vi "Main.vi"() -> ()   [LabVIEW 2021, in "Game of Life.lvlib"]
doc: "This template is for the Queued Message Handler design pattern.\n\nThe Event Handling Loop generates messages based on user interface actions.\n\nThe Message Handling Loop processes messages generated by the Event Handling Loop, or by other messages. The messages are string values, so new messages can be added easily to the Message Cases case structure in the Message Handling Loop. Each message cluster can also provide an optional value for Message Data, which is a variant that can be converted to whatever message-specific data is required."
uses:
  Game of Life.lvlib
  <vilib>/Plug-In SDKs/InstrumentStudio SDK/InstrumentStudioPluginSDK.lvlibp/Plugin Events Enum.ctl
  controls/Data.ctl
  controls/Configuration.ctl
  controls/Game of Life.ctl
  a2cd5499-92a9-455c-b0f9-1db12e3f6067.vi
  aef85ed4-6d5b-4a62-8cd4-232f16e6ae51.vi
  a2cd5499-92a9-455c-b0f9-1db12e3f6067.vi/6651a77e-856e-4bcd-af5a-c0c13b264cc1.vi
  aef85ed4-6d5b-4a62-8cd4-232f16e6ae51.vi/331b549c-fcf8-43d9-8a1e-5b3c0091a99c.vi
  <vilib>/JDP Science/JSONtext/JSON text to Variant.vi
  <vilib>/Utility/error.llb/Error Cluster From Error Code.vi
  <vilib>/JDP Science/JSONtext/Variant to JSON Text.vi
  <vilib>/JDP Science/JSONtext/LVClass Serializer/JSONtext LVClass Serializer.lvclass
  <vilib>/ErrorRing/Error Ring.xnode
  <vilib>/Plug-In SDKs/InstrumentStudio SDK/InstrumentStudioPluginSDK.lvlibp/Plugin Session.lvclass
  <vilib>/Plug-In SDKs/InstrumentStudio SDK/InstrumentStudioPluginSDK.lvlibp
panel:
  in  "Tab Control":enum32{"Game Panel", "Events"}(tab)
  in  "Start":bool
  out "game of life":T1(graph)
  out "generation":u32 caption="Generation"
  in  "update interval":u32=250 caption="Update interval (msec)" min=50
  in  "height":u32=100 caption="Board height" min=10
  in  "width":u32=100 caption="Board width" min=10
  in  "Log Events?":bool
  out "Event Record":i32(listbox)
  in  "Session Id":u64
  # "Enable Logging: Check this box to generate a log file and save the event record."
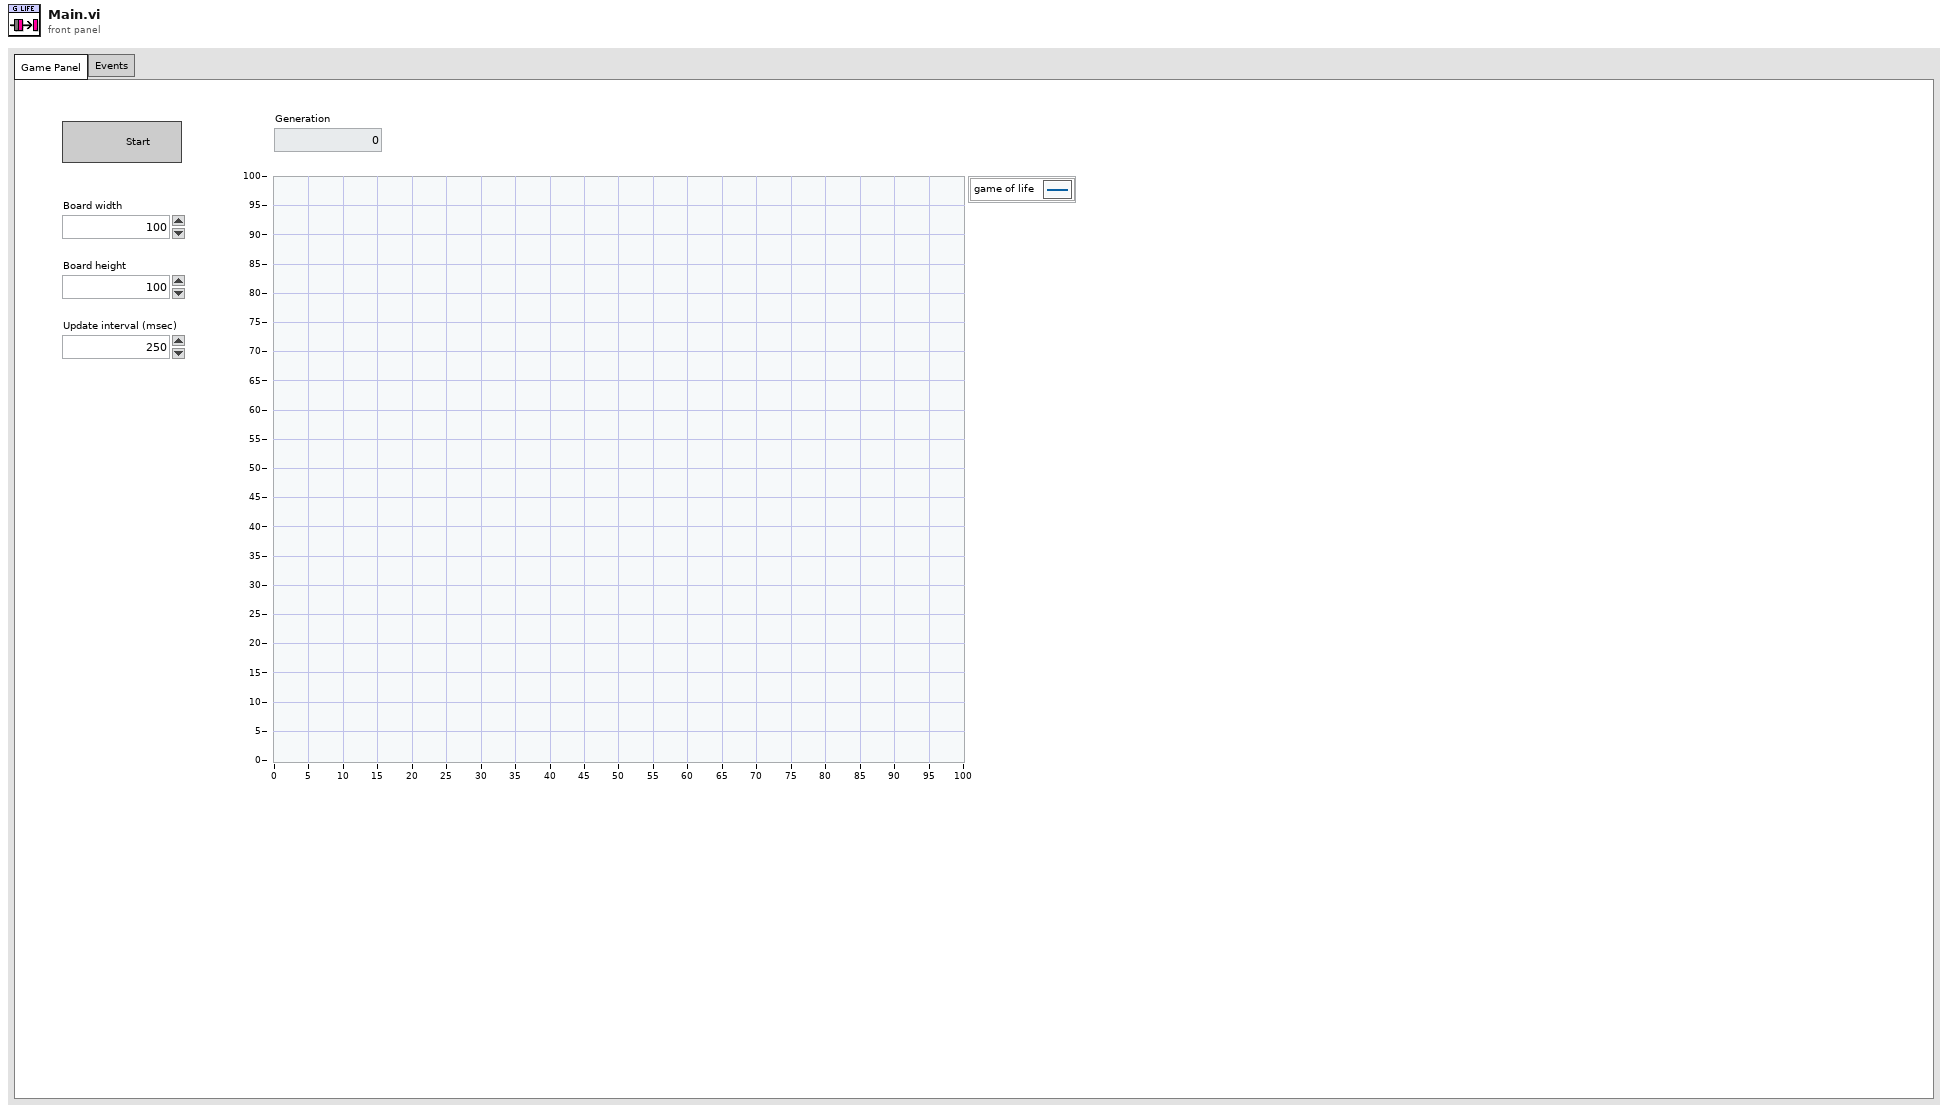
[diagram p1: front panel]
types:
  T1 = typedef "Game of Life.lvlib/Game of Life.ctl" = cluster{"x_data":dbl[], "y_data":dbl[]}
  T2 = typedef "Game of Life.lvlib/Data.ctl" = cluster{"Configuration":T3, "Generation":u32, "Run?":bool, "Cells":bool[][], "Log Events?":bool}
  T3 = typedef "Game of Life.lvlib/Configuration.ctl" = cluster{"Height":u32, "Width":u32, "Update Interval":u32}
  T4 = typedef "InstrumentStudioPluginSDK.lvlibp/Plugin Events Enum.ctl" = enum16{"Shutdown", "Project Saved", "Stop All Outputs"}
  T5 = typedef "InstrumentStudioPluginSDK.lvlibp/Event Registration Refnum.ctl" = refnum<event-registration>
  T6 = typedef "Game of Life.lvlib/All Message Queues.ctl" = cluster{"UI":refnum<queue>}
  T7 = cluster{"Event Refnum":T5, "Event Registration Refnum":refnum<event-registration>}
  T8 = enum8{"Enabled", "Disabled", "Disabled and Grayed Out"}
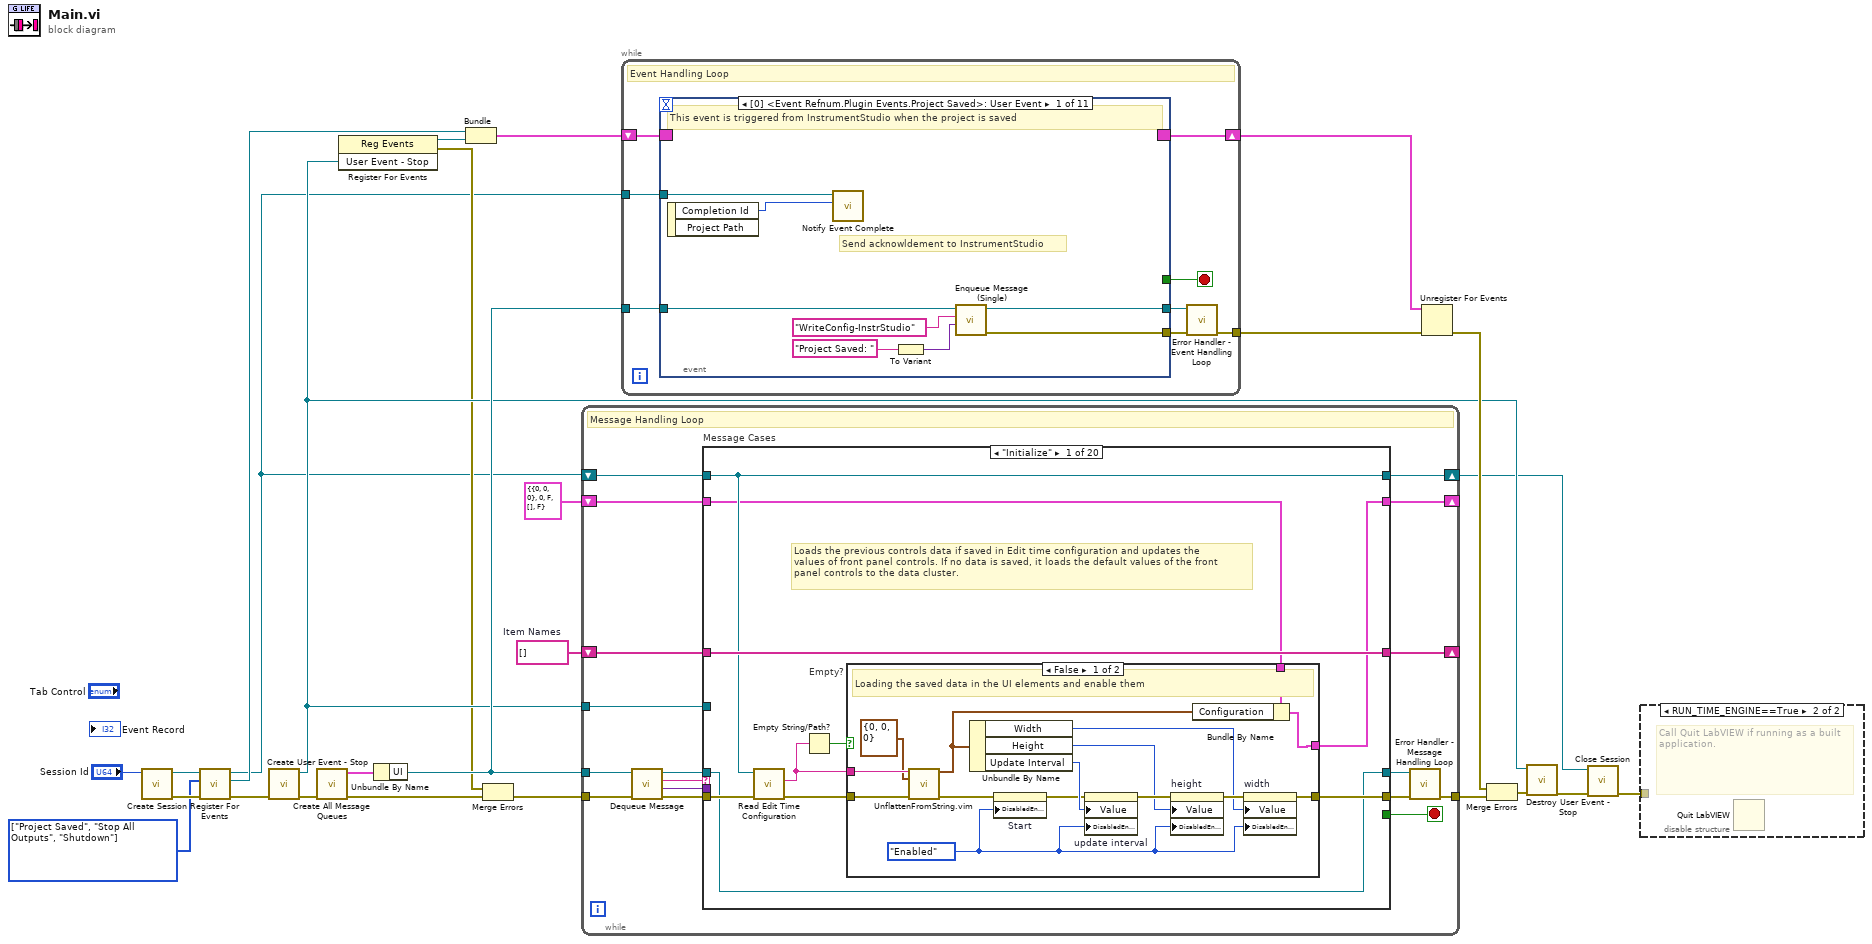
[diagram p0: block diagram]
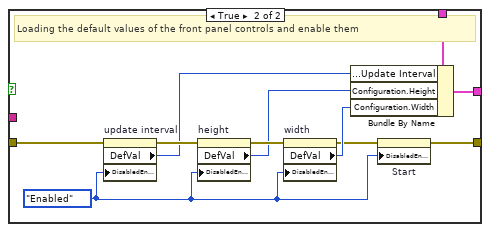
[diagram p3: hidden frame]
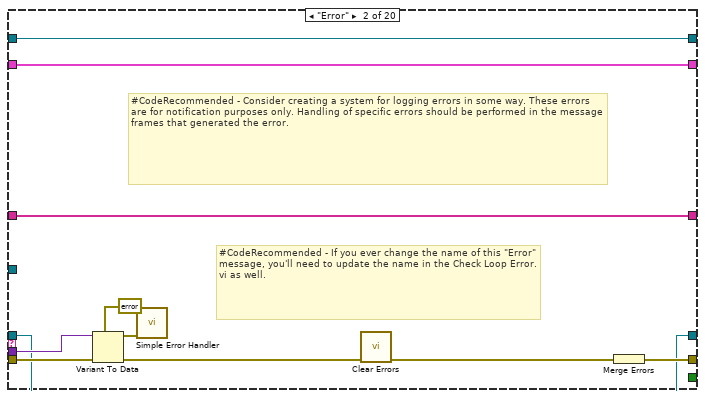
[diagram p4: hidden frame]
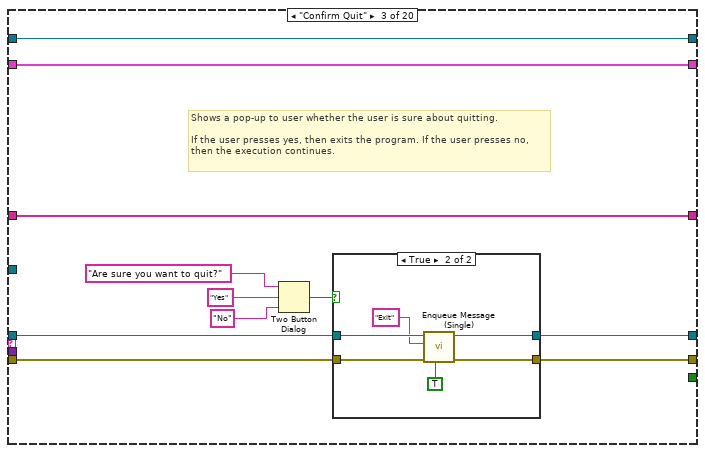
[diagram p5: hidden frame]
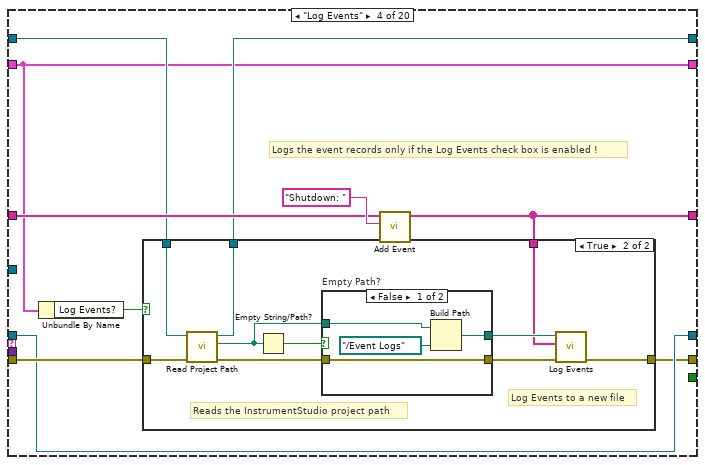
[diagram p7: hidden frame]
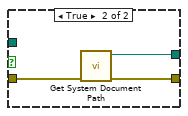
[diagram p9: hidden frame]
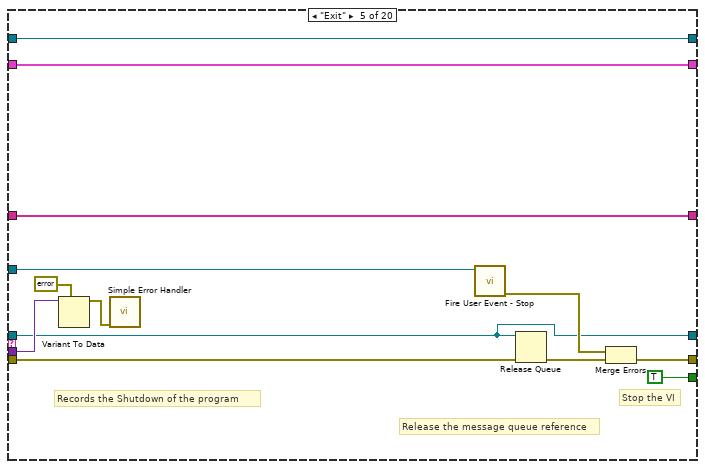
[diagram p10: hidden frame]
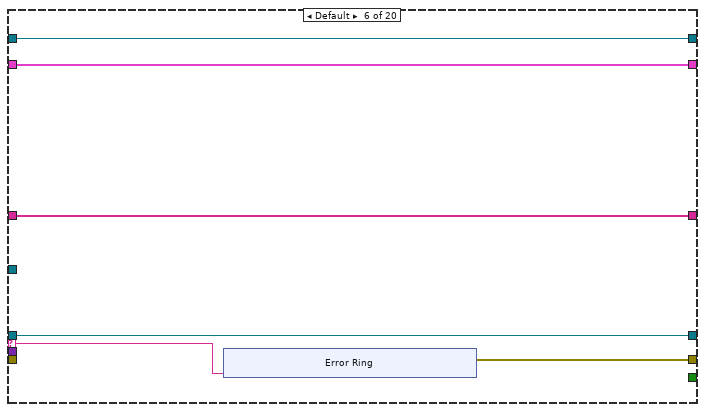
[diagram p11: hidden frame]
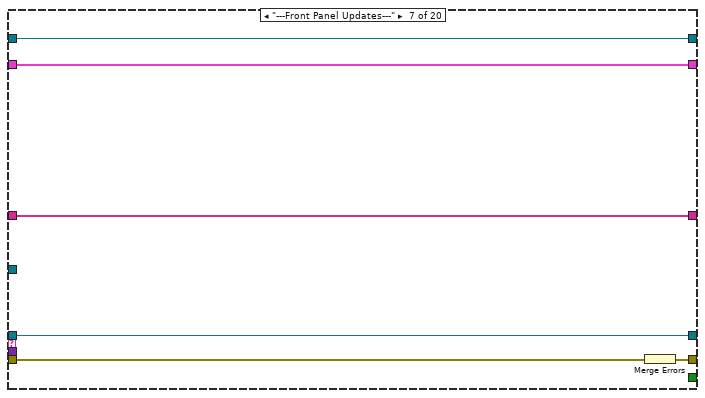
[diagram p12: hidden frame]
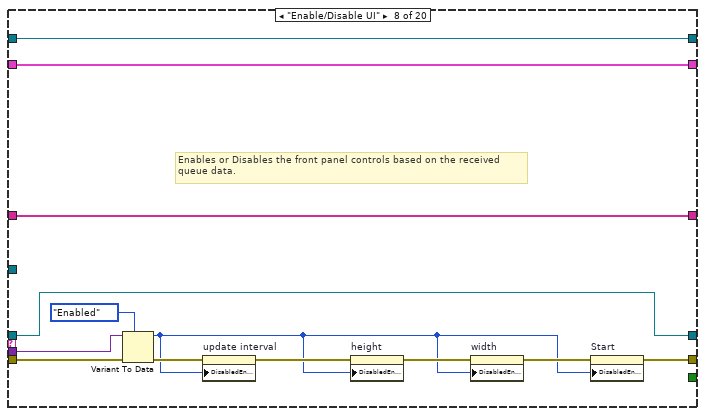
[diagram p13: hidden frame]
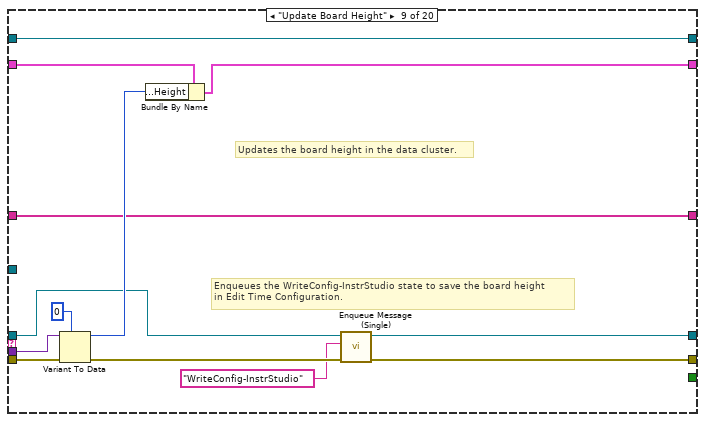
[diagram p14: hidden frame]
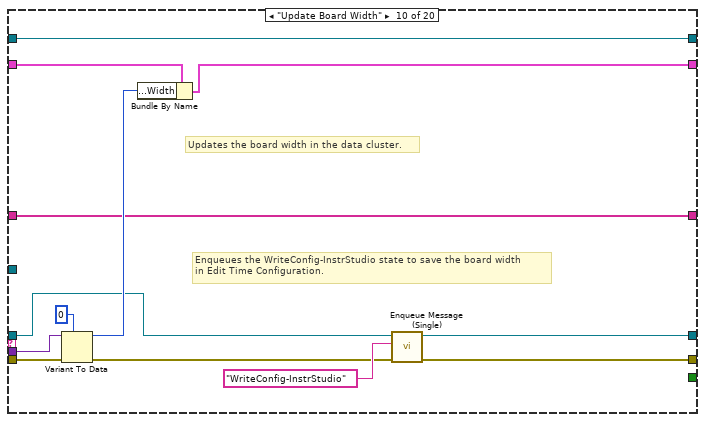
[diagram p15: hidden frame]
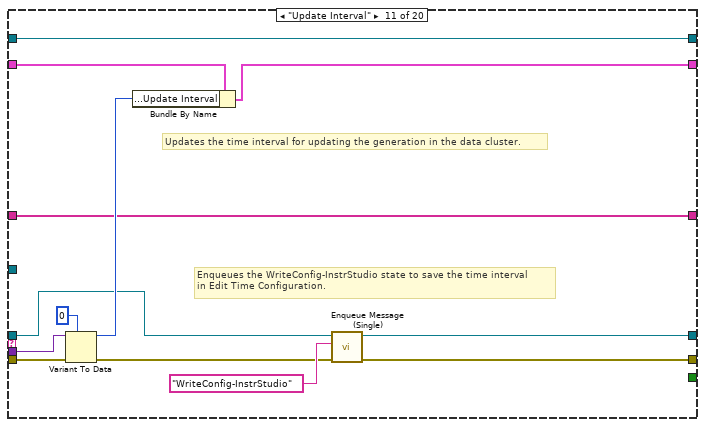
[diagram p16: hidden frame]
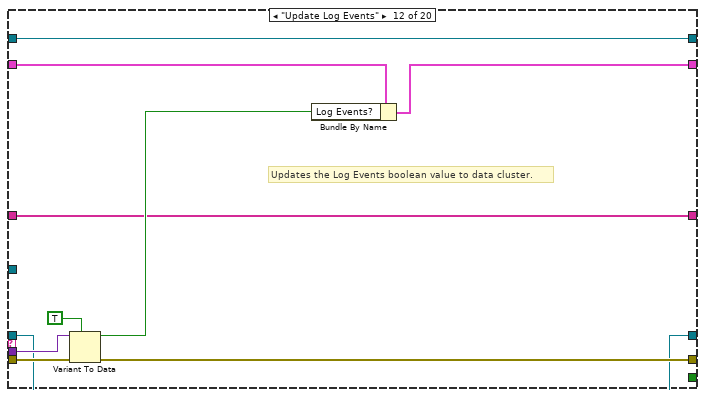
[diagram p17: hidden frame]
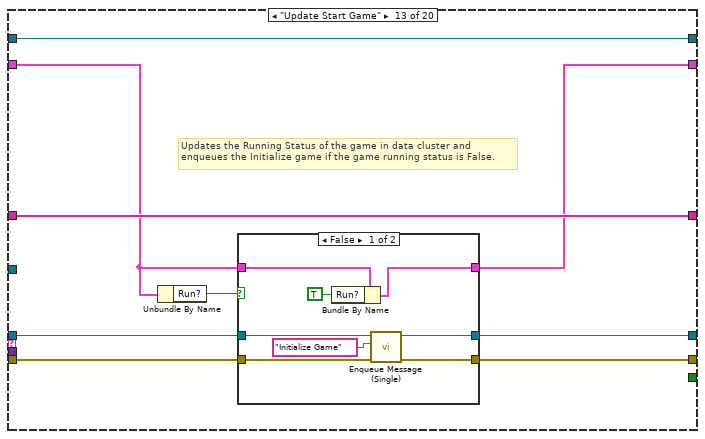
[diagram p18: hidden frame]
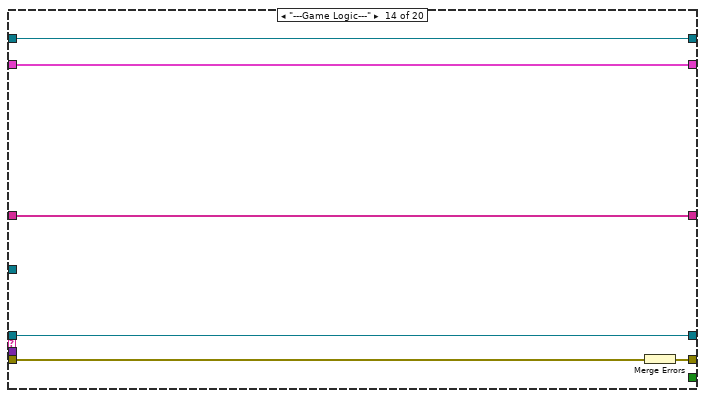
[diagram p20: hidden frame]
diagram:
  w1 = string[] []  # Item Names
  w10 = T4[] [enum."Project Saved", enum."Stop All Outputs", enum."Shutdown"] items=["Shutdown", "Project Saved", "Stop All Outputs"] ("Events To Register")
  n1 = call <vilib>:"Create Session.vi"("Session Id"="Session Id") -> ("error out"=w13:errorcluster, "Session out"=w11:refnum<class "Plugin Session.lvclass">)  [unwired: 6 in, 3 out]
  n2 = call <vilib>:"Register For Events.vi"("error in (no error)"=w13, "Events To Register"=w10, "Session in"=w11) -> ("error out"=w12:errorcluster, "Event Refnum"=w7:T5, "Session out"=w3:refnum<class "Plugin Session.lvclass">)  [unwired: 6 in]
  n3 = call "Create User Event - Stop.vi"("error in (no error)"=w12) -> ("error out"=w22:errorcluster, "User Event - Stop"=w17:refnum<user-event>)  [unwired: 9 in]
  n4 = call "Create All Message Queues.vi"("error in (no error)"=w22) -> ("error out"=w26:errorcluster, "Message Queues out"=w25:T6)  [unwired: 9 in]
  n5 = register-events(w17) -> (reference out=w9:refnum<event-registration>, error out=w15:errorcluster)  [unwired: 2 in]
  n6 = Unbundle By Name(w25) -> ("UI"=w23:refnum<queue>)
  n7 = Bundle("Event Refnum"=w7, "Event Registration Refnum"=w9) -> (w8:T7)  [unwired: 1 in]
  n8 = Merge Errors(w15, w26) -> (w16:errorcluster)
  n9 = while {
    tunnel: w23 -> [w37]
    tunnel: w17 -> [w42]
    tunnel: w16 -> [w41]
    tunnel: [w35] -> w24
    shift-right: [w32] -> w6
    shift-left: w3 -> [w33]
    shift-right: [w31] -> _
    shift-left: T2 {"Configuration"={"Height"=0, "Width"=0, "Update Interval"=0}, "Generation"=0, "Run?"=FALSE, "Cells"=[], "Log Events?"=FALSE} ("Configuration") -> [w30]
    shift-right: [w28] -> _
    shift-left: w1 -> [w29]
    stop <- w43 stop-if-true
    # "Message Handling Loop"
    n10 = call "Dequeue Message.vi"("error in (no error)"=w41, "Message Queue"=w37) -> ("error out"=w40:errorcluster, "Message Data"=w38:variant, "Message"=w39:string, "dup Message Queue"=w36:refnum<queue>)  [unwired: 6 in]
    n11 = case "Message Cases" shown="\"Initialize\"" w39 {
      selector: w39 -> [_ _ _ _ _ w155 _ _ _ _ _ _ _ _ _ _ _ _ _ _]
      tunnel: w36 -> [w46 w80 w99 w114 w140 w151 w164 w171 w184 w197 w209 w226 w233 w252 w271 w284 w318 w334 w343 w355]
      tunnel: w40 -> [w49 w90 w101 w117 w139 _ w169 w175 w194 w207 w220 w229 w239 w257 w269 w289 w323 w336 w345 w354]
      tunnel: [w53 w85 w100 w113 w148 w156 w168 w177 w186 w196 w211 w230 w234 w256 w272 w285 w322 w332 w346 w361] -> w34
      tunnel: [_ _ _ _ TRUE _ _ _ _ _ _ _ _ _ _ _ _ _ _ _] -> w43
      tunnel: w38 -> [_ w89 _ _ w143 _ _ w174 w193 w206 w219 w228 _ _ _ _ _ _ _ w352]
      tunnel: w42 -> [_ _ _ _ w147 _ _ _ _ _ _ _ _ _ _ _ _ _ _ _]
      tunnel: w33 -> [w47 w84 w98 w115 w142 w154 w167 w182 w195 w208 w221 w231 w240 w255 w277 w290 w321 w340 w348 w363]
      tunnel: [w47 w84 w98 w116 w142 w154 w167 w182 w195 w208 w221 w231 w240 w255 w277 w290 w321 w340 w347 w362] -> w32
      tunnel: [w45 w83 w97 w111 w141 w153 w166 w181 w190 w204 w217 w225 w235 w254 w276 w278 w320 w338 w342 w356] -> w31
      tunnel: w30 -> [w44 w83 w97 w111 w141 w153 w166 w181 w189 w203 w216 w224 w236 w254 w275 w282 w320 w337 w342 w356]
      tunnel: w29 -> [w48 w81 w96 w118 w138 w152 w165 w170 w188 w201 w214 w222 w238 w253 w274 w288 w319 w328 w344 w353]
      tunnel: [w48 w81 w96 w112 w138 w152 w165 w170 w188 w201 w214 w222 w238 w253 w274 w288 w319 w329 w344 w357] -> w28
      tunnel: [w46 w80 w95 w114 w140 w151 w164 w171 w185 w198 w210 w226 w232 w252 w270 w281 w318 w330 w343 w355] -> w27
      frame "Initialize" {
        # "Loads the previous controls data if saved in Edit time configuration and updates the\nvalues of front panel controls. If no data is saved, it loads the default values of the front\npanel controls to the data cluster."
        # "Initialize - All initialization work should take place in this message, since other loops can potentially enqueue messages that execute immediately after this one."
        n12 = call <vilib>:"Read Edit Time Configuration.vi"("error in (no error)"=w49, "Session in"=w47) -> ("error out"=w50:errorcluster, "Edit Time Configuration"=w51:string)  [unwired: 7 in, 1 out]
        n13 = Empty String/Path?(string/path=w51) -> (empty?=w52:bool)
        n14 = case "Empty?" shown="False" w52 {
          tunnel: [w62 w70] -> w53
          tunnel: w50 -> [w67 w76]
          tunnel: w51 -> [w68 _]
          tunnel: w44 -> [w59 w79]
          tunnel: [w58 w74] -> w45
          frame False {
            w54 = T8."Enabled" ("Disabled")
            # "Loading the saved data in the UI elements and enable them"
            n15 = call "UnflattenFromString.vim"("Flattened Data"=w68, "Data Type"=T3 {"Height"=0, "Width"=0, "Update Interval"=0} ("Configuration"), "error in"=w67) -> ("Data Out"=w57:T3, "error out"=w56:errorcluster)  [unwired: 11 in]
            n16 = Unbundle By Name(w57) -> ("Width"=w61:u32, "Height"=w64:u32, "Update Interval"=w66:u32)
            n17 = property on="Start" class="Bool"(error in=w56, "DisabledEnum"=w54) -> (error out=w55:errorcluster)  [unwired: 1 in, 1 out]
            n18 = property on="update interval" class="DigNum (strict)"(error in=w55, "Value"=w66, "DisabledEnum"=w54) -> (error out=w65:errorcluster)  [unwired: 1 in, 1 out]
            n19 = property on="height" class="DigNum (strict)"(error in=w65, "Value"=w64, "DisabledEnum"=w54) -> (error out=w63:errorcluster)  [unwired: 1 in, 1 out]
            n20 = Bundle By Name(cluster=w59, "Configuration"=w57) -> (w58:T2)
            n21 = property on="width" class="DigNum (strict)"(error in=w63, "Value"=w61, "DisabledEnum"=w54) -> (error out=w62:errorcluster)  [unwired: 1 in, 1 out]
          }
          frame True {
            w69 = T8."Enabled" ("Disabled")
            # "Loading the default values of the front panel controls and enable them"
            n22 = property on="update interval" class="DigNum (strict)"(error in=w76, "DisabledEnum"=w69) -> (error out=w78:errorcluster, "DefVal"=w75:u32)  [unwired: 1 in, 1 out]
            n23 = property on="height" class="DigNum (strict)"(error in=w78, "DisabledEnum"=w69) -> (error out=w77:errorcluster, "DefVal"=w73:u32)  [unwired: 1 in, 1 out]
            n24 = property on="width" class="DigNum (strict)"(error in=w77, "DisabledEnum"=w69) -> (error out=w71:errorcluster, "DefVal"=w72:u32)  [unwired: 1 in, 1 out]
            n25 = Bundle By Name(cluster=w79, "Configuration.Update Interval"=w75, "Configuration.Height"=w73, "Configuration.Width"=w72) -> (w74:T2)
            n26 = property on="Start" class="Bool"(error in=w71, "DisabledEnum"=w69) -> (error out=w70:errorcluster)  [unwired: 1 in, 1 out]
          }
        }
      }
      frame "Error" {
        # "#CodeRecommended - If you ever change the name of this \"Error\" message, you'll need to update the name in the Check Loop Error.vi as well."
        # "#CodeRecommended - Consider creating a system for logging errors in some way. These errors are for notification purposes only. Handling of specific errors should be performed in the message frames that generated the error."
        # "Error - Display an error dialog. This message is sent by the \"Error Handler\" VIs at the end of other loops in this application."
        n27 = Variant To Data(error in=w90, type=errorcluster {"status"=FALSE, "code"=0, "source"=""} ("error constant"), Variant=w89) -> (data=w87:errorcluster, error out=w86:errorcluster)
        n28 = call <vilib>:"Simple Error Handler.vi"("error in (no error)"=w87) -> ()  [unwired: 4 in, 5 out]
        n29 = call <vilib>:"Clear Errors.vi"("error in (no error)"=w86) -> ("error out"=w82:errorcluster)  [unwired: 5 in, 1 out]
        n30 = Merge Errors(w82) -> (w85:errorcluster)
      }
      frame "Confirm Quit" {
        # "Shows a pop-up to user whether the user is sure about quitting. \n\nIf the user presses yes, then exits the program. If the user presses no,\nthen the execution continues."
        # "Confirm Quit - Message that can confirm whether or not the user wants to exit the application."
        n31 = Two Button Dialog(message="Are sure you want to quit?", 1:"No" ("F button name (\"Cancel\")"), 2:"Yes" ("T button name (\"OK\")")) -> (T button?=w91:bool)
        n32 = case shown="True" w91 {
          tunnel: w101 -> [w102 w109]
          tunnel: [w102 w108] -> w100
          tunnel: w99 -> [w103 w107]
          tunnel: [w103 w104] -> w95
          frame False {
          }
          frame True {
            n33 = call "Enqueue Message (Single).vi"("Priority Message? (F)"=TRUE, "error in (no error)"=w109, "Message"="Exit", "Message Queue"=w107) -> ("error out"=w108:errorcluster, "dup Message Queue"=w104:refnum<queue>)  [unwired: 6 in]
          }
        }
      }
      frame "Log Events" {
        # "Logs the event records only if the Log Events check box is enabled !"
        n34 = Unbundle By Name(w111) -> ("Log Events?"=w110:bool)
        n35 = call "Add Event.vi"("Event Tag"="Shutdown: ", "Item Names in"=w118) -> ("Item Names out"=w112:string[])  [unwired: 9 in]
        n36 = case shown="True" w110 {
          tunnel: w117 -> [w121 w131]
          tunnel: [w120 w130] -> w116
          tunnel: w115 -> [w120 w129]
          tunnel: [w121 w124] -> w113
          tunnel: w112 -> [_ w122]
          frame False {
          }
          frame True {
            # "Log Events to a new file"
            # "Reads the InstrumentStudio project path"
            n37 = call <vilib>:"Read Project Path.vi"("error in (no error)"=w131, "Session in"=w129) -> ("error out"=w127:errorcluster, "Project Path"=w126:path, "Session out"=w130:refnum<class "Plugin Session.lvclass">)  [unwired: 7 in]
            n38 = Empty String/Path?(string/path=w126) -> (empty?=w128:bool)
            n39 = case "Empty Path?" shown="False" w128 {
              tunnel: w127 -> [w135 w136]
              tunnel: w126 -> [w134 _]
              tunnel: [w132 w137] -> w125
              tunnel: [w135 w136] -> w123
              frame False {
                n40 = Build Path(base path=w134, name or relative path=path "../Event Logs") -> (appended path=w132:path)
              }
              frame True {
                n41 = call "Get System Document Path.vi"() -> ("Public Path"=w137:path)  [unwired: 11 in]
              }
            }
            n42 = call "Log Events.vi"("error in"=w123, "Item Names"=w122, "Event Folder Path"=w125) -> ("error out"=w124:errorcluster)  [unwired: 8 in]
          }
        }
      }
      frame "Exit" {
        # "Records the Shutdown of the program"
        # "Stop the VI"
        # "Release the message queue reference"
        # "Exit - Exit the application."
        n43 = Variant To Data(type=errorcluster {"status"=FALSE, "code"=0, "source"=""} ("error constant"), Variant=w143) -> (data=w144:errorcluster)  [unwired: 1 in, 1 out]
        n44 = call <vilib>:"Simple Error Handler.vi"("error in (no error)"=w144) -> ()  [unwired: 4 in, 5 out]
        n45 = call "Fire User Event - Stop.vi"("User Event - Stop"=w147) -> ("error out"=w146:errorcluster)  [unwired: 10 in]
        n46 = Release Queue(queue=w140, error in (no error)=w139) -> (error out=w149:errorcluster)  [unwired: 1 in, 2 out]
        n47 = Merge Errors(w146, w149) -> (w148:errorcluster)
      }
      frame Default {
        # "'Default' case only runs if there is a message that isn't defined in any of the other cases.  Output a programming error."
        n48 = xnode "Error Ring"("parameter 0"=w155) -> ("error out"=w156:errorcluster)
      }
      frame "---Front Panel Updates---" {
        # "Duplicate this frame when creating new messages.  Change this comment in the duplicated frame to describe this message."
        n49 = Merge Errors(w169) -> (w168:errorcluster)
      }
      frame "Enable/Disable UI" {
        # "Enables or Disables the front panel controls based on the received \nqueue data."
        n50 = Variant To Data(error in=w175, type=T8."Enabled" ("Disabled"), Variant=w174) -> (data=w172:T8, error out=w176:errorcluster)
        n51 = property on="update interval" class="DigNum (strict)"(error in=w176, "DisabledEnum"=w172) -> (error out=w180:errorcluster)  [unwired: 1 in, 1 out]
        n52 = property on="height" class="DigNum (strict)"(error in=w180, "DisabledEnum"=w172) -> (error out=w179:errorcluster)  [unwired: 1 in, 1 out]
        n53 = property on="width" class="DigNum (strict)"(error in=w179, "DisabledEnum"=w172) -> (error out=w178:errorcluster)  [unwired: 1 in, 1 out]
        n54 = property on="Start" class="Bool"(error in=w178, "DisabledEnum"=w172) -> (error out=w177:errorcluster)  [unwired: 1 in, 1 out]
      }
      frame "Update Board Height" {
        # "Enqueues the WriteConfig-InstrStudio state to save the board height\nin Edit Time Configuration."
        # "Updates the board height in the data cluster."
        n55 = Variant To Data(error in=w194, type=u32 0 ("wid"), Variant=w193) -> (data=w191:u32, error out=w187:errorcluster)
        n56 = Bundle By Name(cluster=w189, "Configuration.Height"=w191) -> (w190:T2)
        n57 = call "Enqueue Message (Single).vi"("error in (no error)"=w187, "Message"="WriteConfig-InstrStudio", "Message Queue"=w184) -> ("error out"=w186:errorcluster, "dup Message Queue"=w185:refnum<queue>)  [unwired: 7 in]
      }
      frame "Update Board Width" {
        # "Enqueues the WriteConfig-InstrStudio state to save the board width\nin Edit Time Configuration."
        # "Updates the board width in the data cluster."
        n58 = Variant To Data(error in=w207, type=u32 0 ("wid"), Variant=w206) -> (data=w202:u32, error out=w199:errorcluster)
        n59 = Bundle By Name(cluster=w203, "Configuration.Width"=w202) -> (w204:T2)
        n60 = call "Enqueue Message (Single).vi"("error in (no error)"=w199, "Message"="WriteConfig-InstrStudio", "Message Queue"=w197) -> ("error out"=w196:errorcluster, "dup Message Queue"=w198:refnum<queue>)  [unwired: 7 in]
      }
      frame "Update Interval" {
        # "Enqueues the WriteConfig-InstrStudio state to save the time interval\nin Edit Time Configuration."
        # "Updates the time interval for updating the generation in the data cluster."
        n61 = Variant To Data(error in=w220, type=u32 0 ("wid"), Variant=w219) -> (data=w215:u32, error out=w212:errorcluster)
        n62 = Bundle By Name(cluster=w216, "Configuration.Update Interval"=w215) -> (w217:T2)
        n63 = call "Enqueue Message (Single).vi"("error in (no error)"=w212, "Message"="WriteConfig-InstrStudio", "Message Queue"=w209) -> ("error out"=w211:errorcluster, "dup Message Queue"=w210:refnum<queue>)  [unwired: 7 in]
      }
      frame "Update Log Events" {
        # "Updates the Log Events boolean value to data cluster."
        n64 = Variant To Data(error in=w229, type=TRUE, Variant=w228) -> (data=w223:bool, error out=w230:errorcluster)
        n65 = Bundle By Name(cluster=w224, "Log Events?"=w223) -> (w225:T2)
      }
      frame "Update Start Game" {
        # "Updates the Running Status of the game in data cluster and\nenqueues the Initialize game if the game running status is False."
        n66 = Unbundle By Name(w236) -> ("Run?"=w237:bool)
        n67 = case shown="False" w237 {
          tunnel: w239 -> [w243 w250]
          tunnel: w236 -> [w248 w251]
          tunnel: [w247 w251] -> w235
          tunnel: [w244 w250] -> w234
          tunnel: w233 -> [w245 w249]
          tunnel: [w242 w249] -> w232
          frame False {
            n68 = Bundle By Name(cluster=w248, "Run?"=TRUE) -> (w247:T2)
            n69 = call "Enqueue Message (Single).vi"("error in (no error)"=w243, "Message"="Initialize Game", "Message Queue"=w245) -> ("error out"=w244:errorcluster, "dup Message Queue"=w242:refnum<queue>)  [unwired: 7 in]
          }
          frame True {
          }
        }
      }
      frame "---Game Logic---" {
        # "Duplicate this frame when creating new messages.  Change this comment in the duplicated frame to describe this message."
        n70 = Merge Errors(w257) -> (w256:errorcluster)
      }
      frame "Initialize Game" {
        w268 = -1.0 ("X Scale.Range:Minimum")
        # "Generate an initial random \nliving cells in a 2D array"
        # "Initializes the Board"
        n71 = Unbundle By Name(w275) -> ("Configuration.Width"=w266:u32, "Configuration.Height"=w264:u32)
        n72 = To Double Precision Float(number=w266) -> (double precision float=w267:dbl)
        n73 = To Double Precision Float(number=w264) -> (double precision float=w265:dbl)
        n74 = call "Initialize Game.vi"("Height"=w264, "Width"=w266) -> ("Array"=w273:bool[][])  [unwired: 9 in]
        n75 = property on="game of life" class="XYGraph (strict)"(error in=w269, "XScale.Minimum"=w268, "XScale.Maximum"=w267, "YScale.Minimum"=w268, "YScale.Maximum"=w265, "Value"=T1 {"x_data"=[], "y_data"=[]} ("game of life")) -> (error out=w263:errorcluster)  [unwired: 1 in, 1 out]
        n76 = Bundle By Name(cluster=w275, "Generation"=u32 0, "Cells"=w273) -> (w276:T2)
        n77 = call "Enum to Variant Array.vi"("Disabled"=T8."Disabled and Grayed Out") -> ("Message Data Array"=w258:variant[])  [unwired: 10 in]
        n78 = call "Enqueue Message (Array).vi"("error in (no error)"=w263, "Message Data Array"=w258, "Message Array"=string[] ["Enable/Disable UI", "UpdateRunningFlag-InstrStudio", "Game of Life"], "Message Queue"=w271) -> ("error out"=w272:errorcluster, "dup Message Queue"=w270:refnum<queue>)  [unwired: 6 in]
      }
      frame "Game of Life" {
        # "If the stop condition is met, then stops execution of the \ngame logic. If not, keeps executing the game logic by \nenqueueing the present state."
        # "Generates the next generation of living cells by\nappliying game logic to the current generation \nliving cells with the specified time interval."
        n79 = in-place {
          in-place-border: w289 -> [w299]
          in-place-border: [w295] -> w286
          in-place-border: [w294] -> w287
          in-place-border: [w293] -> w283
          in-place-border: [w291] -> w280
          n80 = in-place-cluster #1(w282) -> ("Cells"=w298:bool[][], "Generation"=w297:u32, "Configuration.Update Interval"=w292:u32)
          n81 = call "Wrap Next Generation.vi"("error in"=w299, "Update Interval"=w292, "generation in"=w297, "cells in"=w298) -> ("error out"=w295:errorcluster, "game of life"=w293:T1, "generation out"=w291:u32, "cells out"=w296:bool[][], "Stop?"=w294:bool)  [unwired: 3 in]
          n82 = in-place-cluster #1("Cells"=w296, "Generation"=w291, "Configuration.Update Interval"=w292) -> (w279:T2)
        }
        n83 = case "Stop?" shown="False" w287 {
          tunnel: w286 -> [w304 w313]
          tunnel: [w307 w314] -> w285
          tunnel: w284 -> [w306 w312]
          tunnel: w283 -> [w301 _]
          tunnel: [w303 w311] -> w281
          tunnel: w280 -> [w302 _]
          tunnel: w279 -> [w300 w309]
          tunnel: [w300 w310] -> w278
          frame False {
            n84 = call "Enqueue Message (Single).vi"("error in (no error)"=w304, "Message"="Game of Life", "Message Queue"=w306) -> ("error out"=w307:errorcluster, "dup Message Queue"=w303:refnum<queue>)  [unwired: 7 in]
            "generation" <- w302
            "game of life" <- w301
          }
          frame True {
            n85 = call "Enum to Variant Array.vi"("Disabled"=T8."Enabled") -> ("Message Data Array"=w317:variant[])  [unwired: 10 in]
            n86 = Bundle By Name(cluster=w309, "Run?"=FALSE) -> (w310:T2)
            n87 = call "Enqueue Message (Array).vi"("error in (no error)"=w313, "Message Data Array"=w317, "Message Array"=string[] ["Enable/Disable UI", "UpdateRunningFlag-InstrStudio"], "Message Queue"=w312) -> ("error out"=w314:errorcluster, "dup Message Queue"=w311:refnum<queue>)  [unwired: 6 in]
          }
        }
      }
      frame "---Instrument Studio Interaction---" {
        # "Duplicate this frame when creating new messages.  Change this comment in the duplicated frame to describe this message."
        n88 = Merge Errors(w323) -> (w322:errorcluster)
      }
      frame "StopAllOutputs" {
        # "Flush the Queue to stop game logic execution"
        # "Updates the Running Status of the game in data cluster"
        # "Updates the Event Record indicator with current event."
        n89 = call "Add Event.vi"("Event Tag"="Stop All Outputs: ", "Item Names in"=w328) -> ("Item Names out"=w329:string[])  [unwired: 9 in]
        n90 = property on="Event Record" class="LstBox (strict)"(error in=w336, "Item Names"=w329) -> (error out=w335:errorcluster)  [unwired: 1 in, 1 out]
        n91 = Bundle By Name(cluster=w337, "Run?"=FALSE) -> (w338:T2)
        n92 = Flush Queue(queue=w334, error in (no error)=w335) -> (queue out=w331:refnum<queue>, error out=w333:errorcluster)  [unwired: 1 out]
        n93 = call "Enum to Variant Array.vi"("Disabled"=T8."Enabled") -> ("Message Data Array"=w325:variant[])  [unwired: 10 in]
        n94 = call "Enqueue Message (Array).vi"("error in (no error)"=w333, "Message Data Array"=w325, "Message Array"=string[] ["Enable/Disable UI", "UpdateRunningFlag-InstrStudio"], "Message Queue"=w331) -> ("error out"=w332:errorcluster, "dup Message Queue"=w330:refnum<queue>)  [unwired: 6 in]
      }
      frame "UpdateRunningFlag-InstrStudio" {
        # "Updates the running flag in \nInstrumentStudio"
        n95 = Unbundle By Name(w342) -> ("Run?"=w341:bool)
        n96 = call <vilib>:"Update Running State.vi"("error in (no error)"=w345, "Is Running"=w341, "Plugin Session in"=w348) -> ("error out"=w346:errorcluster, "Plugin Session out"=w347:refnum<class "Plugin Session.lvclass">)  [unwired: 7 in]
      }
      frame "WriteConfig-InstrStudio" {
        # "Saving the control inputs\nin the instrumentStudio object"
        n97 = Equal?(x=w352, y=variant) -> (x = y?=w350:bool)
        n98 = case "Empty Variant?" shown="False" w350 {
          tunnel: [w371 w372] -> w358
          tunnel: [w370 w373] -> w357
          tunnel: w354 -> [w366 w372]
          tunnel: w352 -> [w365 _]
          tunnel: w353 -> [w369 w373]
          frame False {
            # "Records the project save event in event record indicator."
            n99 = Variant To Data(error in=w366, type="", Variant=w365) -> (data=w364:string, error out=w367:errorcluster)
            n100 = call "Add Event.vi"("Event Tag"=w364, "Item Names in"=w369) -> ("Item Names out"=w370:string[])  [unwired: 9 in]
            n101 = property on="Event Record" class="LstBox (strict)"(error in=w367, "Item Names"=w370) -> (error out=w371:errorcluster)  [unwired: 1 in, 1 out]
          }
          frame True {
          }
        }
        n102 = Unbundle By Name(w356) -> ("Configuration"=w349:T3)
        n103 = call "FlattenToString.vim"("Anything"=w349, "error in"=w358) -> ("Flattened Data"=w360:string, "error out"=w359:errorcluster)  [unwired: 12 in]
        n104 = call <vilib>:"Write Edit Time Configuration.vi"("error in (no error)"=w359, "Edit Time Configuration"=w360, "Session in"=w363) -> ("error out"=w361:errorcluster, "Session out"=w362:refnum<class "Plugin Session.lvclass">)  [unwired: 7 in]
      }
    }
    n105 = call "Error Handler - Message Handling Loop.vi"("error in (no error)"=w34, "Message Queue"=w27) -> ("dup error in"=w35:errorcluster)  [unwired: 8 in, 1 out]
  }
  n106 = while {
    tunnel: w23 -> [w381]
    shift-right: [w379] -> w19
    shift-left: w8 -> [w380]
    tunnel: [w375] -> w18
    tunnel: w3 -> [w374]
    stop <- w377 stop-if-true
    # "Event Handling Loop"
    n107 = event shown="[0] <Event Refnum.Plugin Events.Project Saved>: User Event" {
      selector: w380 -> [_ _ _ _ _ _ _ _ _ _ _]
      dyn-events: [_ _ _ _ _ _ _ _ _ _ _] -> w379
      timeout: _ -> [_ _ _ _ _ _ _ _ _ _ _]
      tunnel: [_ _ _ _ _ _ _ _ _ _ TRUE ("Discard?")] -> w377
      tunnel: w381 -> [w386 w394 w399 w405 w411 w417 w422 w426 w433 w435 w437]
      tunnel: [w384 w391 w400 w404 w410 w416 _ w425 w432 _ _] -> w378
      tunnel: [w385 w392 w401 w406 w412 w418 w421 w427 w431 w435 w437] -> w376
      tunnel: w374 -> [w389 w396 _ _ _ _ _ _ _ _ _]
      event User Event {
        # "Send acknowldement to InstrumentStudio"
        # "This event is triggered from InstrumentStudio when the project is saved"
        n108 = event-data() -> ("Completion Id"=w388:i64)  [unwired: 1 in, 1 out]
        n109 = call <vilib>:"Notify Event Complete.vi"("Completion Id"=w388, "Session in"=w389) -> ()  [unwired: 8 in, 2 out]
        n110 = To Variant(anything="Project Saved: " ("string")) -> (Variant=w383:variant)
        n111 = call "Enqueue Message (Single).vi"("Message Data"=w383, "Message"="WriteConfig-InstrStudio", "Message Queue"=w386) -> ("error out"=w384:errorcluster, "dup Message Queue"=w385:refnum<queue>)  [unwired: 7 in]
      }
      event User Event {
        # "Send acknowldement to InstrumentStudio"
        # "This event is triggered from InstrumentStudio when the project Stop All Outputs button is pressed"
        n112 = event-data() -> ("Completion Id"=w395:i64)  [unwired: 1 in]
        n113 = call <vilib>:"Notify Event Complete.vi"("Completion Id"=w395, "Session in"=w396) -> ()  [unwired: 8 in, 2 out]
        n114 = call "Enqueue Message (Single).vi"("Priority Message? (F)"=TRUE, "Message"="StopAllOutputs", "Message Queue"=w394) -> ("error out"=w391:errorcluster, "dup Message Queue"=w392:refnum<queue>)  [unwired: 7 in]
      }
      event User Event {
        # "This event doesn't need acknowledgement from plugin"
        # "This event is triggered when softpanel/instrumentstudio is closed"
        n115 = event-data() -> ()  [unwired: 1 in, 1 out]
        n116 = call "Enqueue Message (Array).vi"("Priority Message? Array"=bool[] [TRUE, TRUE], "Message Array"=string[] ["Log Events", "Exit"], "Message Queue"=w399) -> ("error out"=w400:errorcluster, "dup Message Queue"=w401:refnum<queue>)  [unwired: 7 in]
      }
      event "height": Value Change {
        # "Captures value change in height and sends data to Message Handling Loop"
        n117 = event-data() -> ("NewVal"=w403:u32)  [unwired: 1 in]
        n118 = To Variant(anything=w403) -> (Variant=w402:variant)
        n119 = call "Enqueue Message (Single).vi"("Message Data"=w402, "Message"="Update Board Height", "Message Queue"=w405) -> ("error out"=w404:errorcluster, "dup Message Queue"=w406:refnum<queue>)  [unwired: 7 in]
      }
      event "width": Value Change {
        # "Captures value change in width and sends data to Message Handling Loop"
        n120 = event-data() -> ("NewVal"=w409:u32)  [unwired: 1 in]
        n121 = To Variant(anything=w409) -> (Variant=w408:variant)
        n122 = call "Enqueue Message (Single).vi"("Message Data"=w408, "Message"="Update Board Width", "Message Queue"=w411) -> ("error out"=w410:errorcluster, "dup Message Queue"=w412:refnum<queue>)  [unwired: 7 in]
      }
      event "update interval": Value Change {
        # "Captures value change in update interval and sends data to Message Handling Loop"
        n123 = event-data() -> ("NewVal"=w415:u32)  [unwired: 1 in]
        n124 = To Variant(anything=w415) -> (Variant=w414:variant)
        n125 = call "Enqueue Message (Single).vi"("Message Data"=w414, "Message"="Update Interval", "Message Queue"=w417) -> ("error out"=w416:errorcluster, "dup Message Queue"=w418:refnum<queue>)  [unwired: 7 in]
      }
      event "Log Events?": Value Change {
        # "Captures value change in Log Events and sends data to Message Handling Loop"
        n126 = event-data() -> ("NewVal"=w420:bool)  [unwired: 1 in]
        n127 = To Variant(anything=w420) -> (Variant=w423:variant)
        n128 = call "Enqueue Message (Single).vi"("Message Data"=w423, "Message"="Update Log Events", "Message Queue"=w422) -> ("dup Message Queue"=w421:refnum<queue>)  [unwired: 7 in, 1 out]
      }
      event "Start": Value Change {
        # "Captures value change in height and enqueues a state for Message Handling Loop"
        n129 = event-data() -> ()  [unwired: 1 in, 1 out]
        n130 = call "Enqueue Message (Single).vi"("Message"="Update Start Game", "Message Queue"=w426) -> ("error out"=w425:errorcluster, "dup Message Queue"=w427:refnum<queue>)  [unwired: 8 in]
      }
      event Panel Close? {
        # "Send the 'Confirm Quit' message if the user closes the panel of the VI. Discard the event so the 'Confirm Quit' message has a chance to run."
        n131 = event-data() -> ()  [unwired: 1 in, 1 out]
        n132 = call-poly "Enqueue Message.vi"("Priority Message? (F)"=TRUE, "Message"="Confirm Quit", "Message Queue"=w433) -> ("error out"=w432:errorcluster, "dup Message Queue"=w431:refnum<queue>)  [unwired: 7 in]
        n133 = event-data("Discard?"=TRUE) -> ()  [unwired: 1 in, 1 out]
      }
      event Application Instance Close {
        # "#CodeRecommended - When a project closes, all VIs within that project are aborted and leave memory. However, any code placed in this event frame is guaranteed to run to completion, so add any cleanup code that absolutely must happen here."
        n134 = event-data() -> ()  [unwired: 1 in, 1 out]
      }
      event User Event {
        # "The Message Handling Loop processed an \"Exit\" message, which fired this event to stop the Event Handling Loop."
        n135 = event-data() -> ()  [unwired: 1 in, 1 out]
      }
    }
    n136 = call "Error Handler - Event Handling Loop.vi"("error in (no error)"=w378, "Message Queue"=w376) -> ("dup error in"=w375:errorcluster)  [unwired: 8 in, 1 out]
  }
  n137 = Unregister For Events(event registration refnum=w19, error in=w18) -> (error out=w20:errorcluster)
  n138 = Merge Errors(w20, w24) -> (w21:errorcluster)
  n139 = call "Destroy User Event - Stop.vi"("error in (no error)"=w21, "User Event - Stop"=w17) -> ("error out"=w5:errorcluster)  [unwired: 9 in]
  n140 = call <vilib>:"Close Session.vi"("error in (no error)"=w5, "Session in"=w6) -> ("error out"=w4:errorcluster)  [unwired: 9 in]
  n141 = disable-structure shown="RUN_TIME_ENGINE==True" {
    disable-tunnel: w4 -> [_ _]
    frame condition #0 (active) {
    }
    frame condition #1 {
      # "Call Quit LabVIEW if running as a built application."
      n142 = Quit LabVIEW() -> ()  [unwired: 1 in]
    }
  }
